vi "Do Core.vi"(8 "error in (no error)":errorcluster, 10 "Actor in":refnum<class "Actor.lvclass">, 11 "Message":refnum<class "Post Iteration Msg.lvclass">) -> (0 "error out":errorcluster, 2 "Actor out":refnum<class "Actor.lvclass">, 3 "Iterate":bool)   [LabVIEW 2023, in "Example Iterator NR Actor Implicit Iteration.lvlib" / "Post Iteration Msg.lvclass"]
doc: "(<B>Filename</B>: Actor Framework.lvlib:Reply Msg.lvclass:Do Core.vi)\n\nDefines what an actor does when it receives <B>Reply Message</B>. This method also defines the <B>Reply</B> that is returned to the actor that sent <B>Reply Message</B>.\n\nBy default, this method does nothing, and <B>Reply</B> is the ancestor Message class. A child class must override this method to define behavior and specify a child of the Message class to return in the <B>Reply</B> output."
uses:
  Post Iteration Msg.lvclass
  <vilib>/ActorFramework/Actor/Actor.lvclass
  Example Actor/Example Actor.lvclass
  C:/Program Files/National Instruments/LabVIEW 2023/vi.lib/ActorFramework/Actor/Actor.lvclass
  Post Iteration Msg.lvclass/Post Iteration Msg.ctl
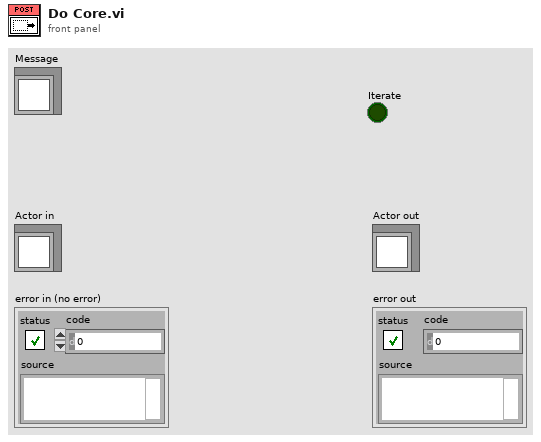
[diagram p1: front panel]
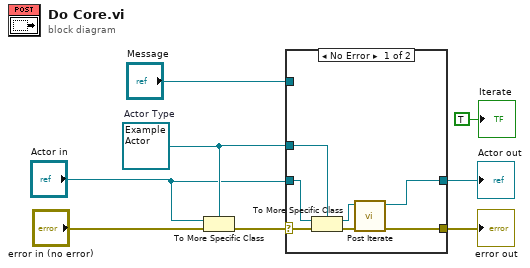
[diagram p0: block diagram]
diagram:
  w3 = refnum<class "Example Actor.lvclass"> refnum  # Actor Type
  n1 = To More Specific Class(target class=w3, reference="Actor in", error in="error in (no error)") -> (error out=w7:errorcluster)  [unwired: 1 out]
  n2 = case shown="No Error" w7 {
    selector: w7 -> [w15 w17]
    tunnel: [w11 w17] -> w4
    tunnel: [w10 w16] -> w5
    tunnel: "Actor in" -> [w14 w16]
    tunnel: w3 -> [w13 _]
    tunnel: "Message" -> [_ _]
    frame No Error {
      n3 = To More Specific Class ("Actor Cast")(target class=w13, reference=w14, error in=w15) -> (specific class reference=w9:refnum<class "Example Actor.lvclass">, error out=w12:errorcluster)
      n4 = call "Post Iterate.vi"("error in (no error)"=w12, "Example Actor in"=w9) -> ("error out"=w11:errorcluster, "Example Actor out"=w10:refnum<class "Example Actor.lvclass">)  [unwired: 8 in]
    }
    frame Error {
    }
  }
  "error out" <- w4
  "Actor out" <- w5
  "Iterate" <- TRUE ("Iterate")
